vi "Shutdown.vi"(8 "Image Processing Loop":errorcluster, 9 "Manipulator Loop":errorcluster, 11 "IO Cluster In":T1={"Error"={"status"=FALSE, "code"=0, "source"=""}, "Encoder Calibration Values"=[22, 216], "Update Calibration"=FALSE, "JPEG Resolutions"=3, "Raw Resolutions"=1, "Image Mode"=enum."RAW Gray Scale", "FPGA Ref"=refnum} {"JPEG Resolutions" items=["160x128"=3, "320x240"=5, "640x480"=7]; "Raw Resolutions" items=["80x60"=1, "160x120"=3, "128x128"=9, "128x96"=11]}) -> (0 "Error":errorcluster)   [LabVIEW 2019]
uses:
  QNET MS IO Cluster.ctl
  <vilib>/Utility/error.llb/Error Cluster From Error Code.vi
  <vilib>/rvi/errors/niLvFpgaAdjustHostInterfaceError.vi
  <vilib>/rvi/interface/nirviReadWriteControl/nirviReadWriteControl.xnode
  NiFpgaLv.dll
  <vilib>/rvi/interface/Simulation/niFpgaSimulationCallBeginRW.vi
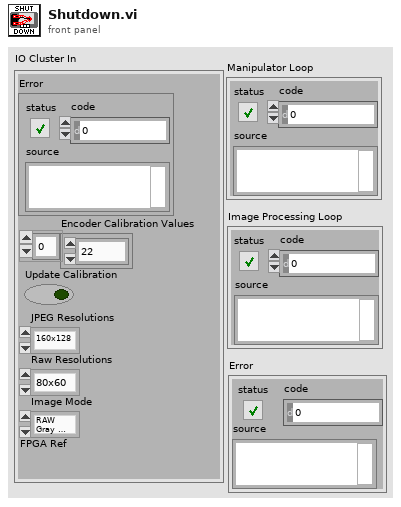
[diagram p1: front panel]
types:
  T1 = typedef "QNET MS IO Cluster.ctl" = cluster{"Error":errorcluster, "Encoder Calibration Values":i32[], "Update Calibration":bool, "JPEG Resolutions":u16, "Raw Resolutions":u16, "Image Mode":enum16{"RAW RGB", "RAW Gray Scale", "JPEG"}, "FPGA Ref":refnum<k20>}
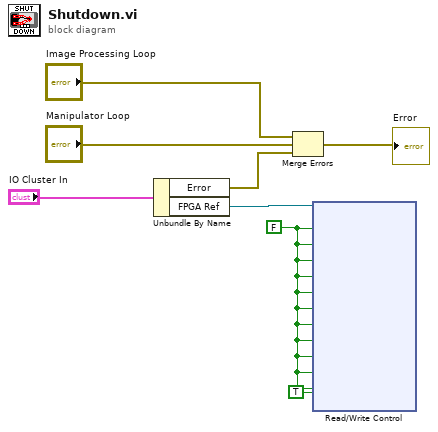
[diagram p0: block diagram]
diagram:
  w8 = FALSE ("PWM0 Enable")
  n1 = Unbundle By Name("IO Cluster In") -> ("Error"=w6:errorcluster, "FPGA Ref"=w7:refnum<k20>)
  n2 = Merge Errors("Image Processing Loop", "Manipulator Loop", w6) -> (→"Error":errorcluster)
  n3 = xnode "Read/Write Control"("FPGA VI引用输入"=w7, "PWM0 Enable"=w8, "PWM1 Enable"=w8, "LED1 Red"=w8, "LED1 Yellow"=w8, "LED1 Green"=w8, "LED2 Red"=w8, "LED2 Yellow"=w8, "LED2 Green"=w8, "LED3 Red"=w8, "LED3 Yellow"=w8, "LED3 Green"=w8, "Camera Power"=TRUE) -> ()  [unwired: 1 in, 2 out]
